vi "Set Session Property.vi"   [LabVIEW 2020, in "SLSC.lvlib"]
uses:
  <vilib>/SLSC/SLSC.lvlib
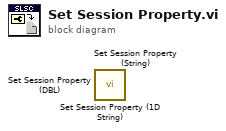
[diagram p0: block diagram]
diagram:
  n1 = call <vilib>:"Set Session Property (1D String).vi"() -> ()  [unwired: 14 in, 2 out]
  n2 = call <vilib>:"Set Session Property (String).vi"() -> ()  [unwired: 14 in, 2 out]
  n3 = call <vilib>:"Set Session Property (DBL).vi"() -> ()  [unwired: 14 in, 2 out]
